vi "Byte177_188 (SubVI).vi"(2 "Channel Number":dbl, 3 "Input String":string) -> (0 "Output Lockout Status":bool, 1 "Output over current alert Ch I2T Levels":T1)   [LabVIEW 2024]
panel:
  in  "Channel Number 2":dbl
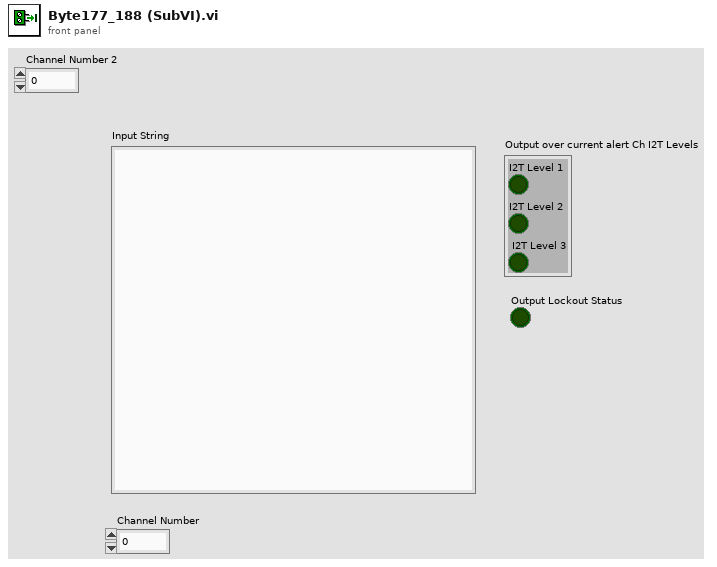
[diagram p1: front panel]
types:
  T1 = cluster{"I2T Level 1":bool, "I2T Level 2":bool, " I2T Level 3":bool}
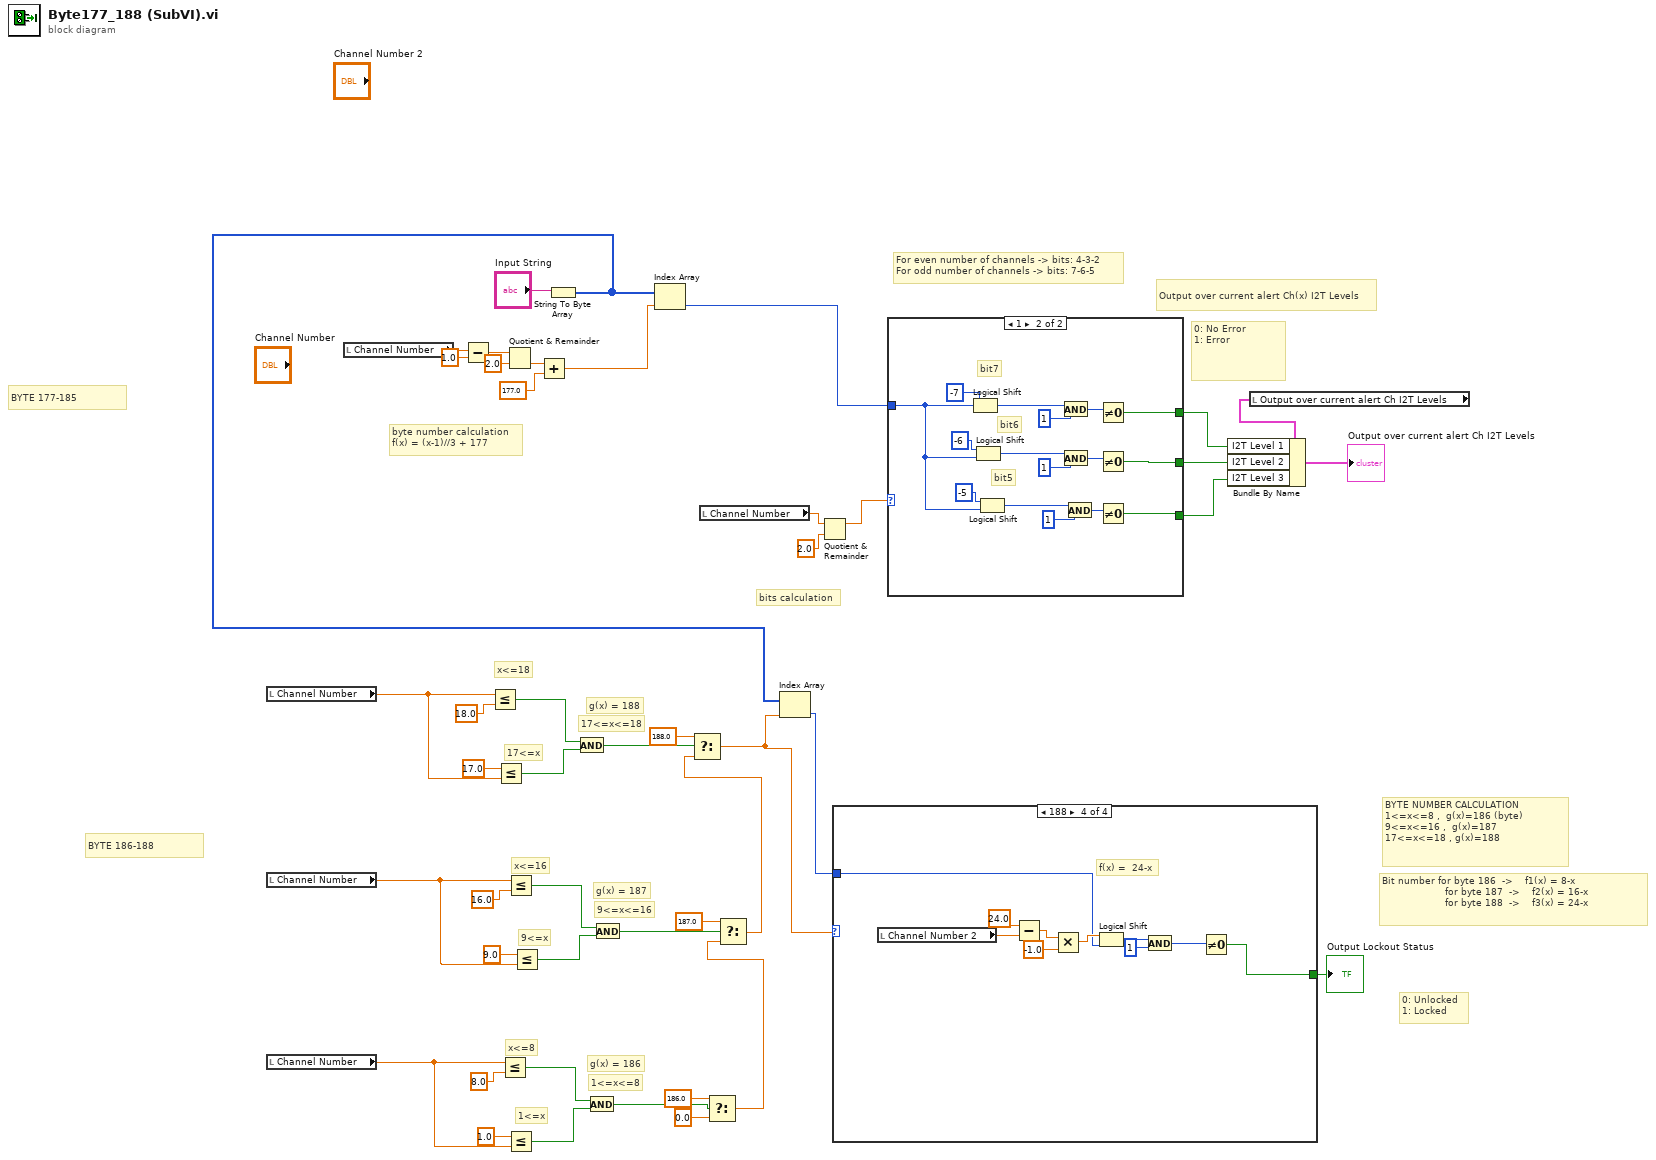
[diagram p0: block diagram]
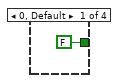
[diagram p2: hidden frame]
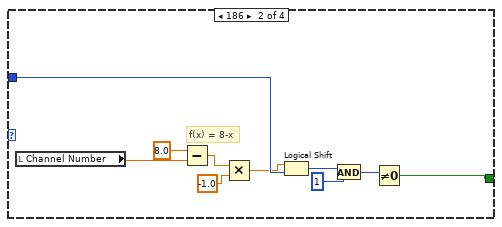
[diagram p3: hidden frame]
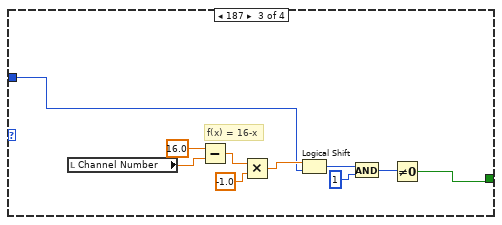
[diagram p4: hidden frame]
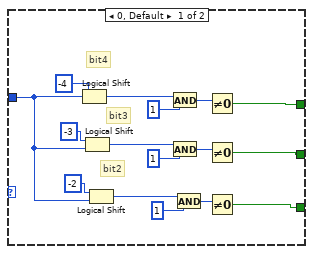
[diagram p5: hidden frame]
diagram:
  # "0: Unlocked\n1: Locked"
  # "BYTE 177-185"
  # "BYTE 186-188"
  # "Bit number for byte 186  ->    f1(x) = 8-x\n                     for byte 187  ->    f2(x) = 16-x\n                     for byte 188  ->    f3(x) = 24-x"
  # "BYTE NUMBER CALCULATION\n1<=x<=8 ,  g(x)=186 (byte)\n9<=x<=16 ,  g(x)=187\n17<=x<=18 , g(x)=188"
  # "g(x) = 186"
  # "1<=x<=8"
  # "1<=x"
  # "x<=8"
  # "g(x) = 187"
  # "g(x) = 188"
  # "9<=x<=16"
  # "9<=x"
  # "x<=16"
  # "17<=x<=18"
  # "17<=x"
  # "x<=18"
  # "byte number calculation\nf(x) = (x-1)//3 + 177"
  # "For even number of channels -> bits: 4-3-2\nFor odd number of channels -> bits: 7-6-5"
  # "0: No Error\n1: Error"
  # "Output over current alert Ch(x) I2T Levels"
  # "bits calculation"
  n1 = local read "Channel Number"() -> (w8:dbl)
  n2 = local read "Channel Number"() -> (w7:dbl)
  n3 = local read "Channel Number"() -> (w6:dbl)
  n4 = local read "Channel Number"() -> (w35:dbl)
  n5 = Subtract(x=w35, y=1.0) -> (x-y=w33:dbl)
  n6 = Less Or Equal?(x=w8, y=18.0) -> (x <= y?=w26:bool)
  n7 = Less Or Equal?(x=17.0, y=w8) -> (x <= y?=w25:bool)
  n8 = Less Or Equal?(x=w6, y=8.0) -> (x <= y?=w18:bool)
  n9 = Quotient & Remainder(x=w33, y=2.0) -> (floor(x/y)=w31:dbl)  [unwired: 1 out]
  n10 = Less Or Equal?(x=w7, y=16.0) -> (x <= y?=w22:bool)
  n11 = Less Or Equal?(x=1.0, y=w6) -> (x <= y?=w17:bool)
  n12 = Less Or Equal?(x=9.0, y=w7) -> (x <= y?=w21:bool)
  n13 = Add(x=w31, y=177.0) -> (x+y=w29:dbl)
  n14 = String To Byte Array(string="Input String") -> (unsigned byte array=w4:u8[])
  n15 = And(x=w26, y=w25) -> (x .and. y?=w16:bool)
  n16 = And(x=w18, y=w17) -> (x .and. y?=w14:bool)
  n17 = And(x=w22, y=w21) -> (x .and. y?=w15:bool)
  n18 = Index Array "Index Array"(array=w4, index=w29) -> (element=w41:u8)
  n19 = local read "Channel Number"() -> (w44:dbl)
  n20 = Select(t=186.0, s=w14, f=0.0) -> (s? t:f=w9:dbl)
  n21 = Select(t=187.0, s=w15, f=w9) -> (s? t:f=w5:dbl)
  n22 = Select(t=188.0, s=w16, f=w5) -> (s? t:f=w1:dbl)
  n23 = Index Array "Index Array"(array=w4, index=w1) -> (element=w2:u8)
  n24 = Quotient & Remainder(x=w44, y=2.0) -> (x-y*floor(x/y)=w42:dbl)  [unwired: 1 out]
  n25 = case shown="188" w1 {
    tunnel: w2 -> [_ w49 w57 w71]
    tunnel: [FALSE w50 w60 w67] -> w3
    frame 0, Default {
    }
    frame 186 {
      # "f(x) = 8-x"
      n26 = local read "Channel Number"() -> (w47:dbl)
      n27 = Subtract(x=8.0, y=w47) -> (x-y=w55:dbl)
      n28 = Multiply(x=w55, y=-1.0) -> (x*y=w48:dbl)
      n29 = Logical Shift(y=w48, x=w49) -> (x << y=w52:u8)
      n30 = And(x=w52, y=u8 1) -> (x .and. y?=w51:u8)
      n31 = Not Equal To 0?(x=w51) -> (x != 0?=w50:bool)
    }
    frame 187 {
      # "f(x) = 16-x"
      n32 = local read "Channel Number"() -> (w58:dbl)
      n33 = Subtract(x=16.0, y=w58) -> (x-y=w64:dbl)
      n34 = Multiply(x=w64, y=-1.0) -> (x*y=w59:dbl)
      n35 = Logical Shift(y=w59, x=w57) -> (x << y=w65:u8)
      n36 = And(x=w65, y=u8 1) -> (x .and. y?=w66:u8)
      n37 = Not Equal To 0?(x=w66) -> (x != 0?=w60:bool)
    }
    frame 188 {
      # "f(x) =  24-x"
      n38 = local read "Channel Number 2"() -> (w76:dbl)
      n39 = Subtract(x=24.0, y=w76) -> (x-y=w74:dbl)
      n40 = Multiply(x=w74, y=-1.0) -> (x*y=w72:dbl)
      n41 = Logical Shift(y=w72, x=w71) -> (x << y=w70:u8)
      n42 = And(x=w70, y=u8 1) -> (x .and. y?=w68:u8)
      n43 = Not Equal To 0?(x=w68) -> (x != 0?=w67:bool)
    }
  }
  "Output Lockout Status" <- w3
  n44 = case shown="1" w42 {
    tunnel: w41 -> [w80 w96]
    tunnel: [w79 w95] -> w39
    tunnel: [w78 w94] -> w40
    tunnel: [w77 w93] -> w38
    frame 0, Default {
      # "bit2"
      # "bit3"
      # "bit4"
      n45 = Logical Shift(y=i16 -4, x=w80) -> (x << y=w89:u8)
      n46 = Logical Shift(y=i16 -3, x=w80) -> (x << y=w85:u8)
      n47 = Logical Shift(y=i16 -2, x=w80) -> (x << y=w84:u8)
      n48 = And(x=w89, y=u8 1) -> (x .and. y?=w91:u8)
      n49 = And(x=w85, y=u8 1) -> (x .and. y?=w86:u8)
      n50 = And(x=w84, y=u8 1) -> (x .and. y?=w83:u8)
      n51 = Not Equal To 0?(x=w91) -> (x != 0?=w79:bool)
      n52 = Not Equal To 0?(x=w86) -> (x != 0?=w78:bool)
      n53 = Not Equal To 0?(x=w83) -> (x != 0?=w77:bool)
    }
    frame 1 {
      # "bit5"
      # "bit6"
      # "bit7"
      n54 = Logical Shift(y=i16 -7, x=w96) -> (x << y=w105:u8)
      n55 = Logical Shift(y=i16 -6, x=w96) -> (x << y=w101:u8)
      n56 = Logical Shift(y=i16 -5, x=w96) -> (x << y=w100:u8)
      n57 = And(x=w105, y=u8 1) -> (x .and. y?=w107:u8)
      n58 = And(x=w101, y=u8 1) -> (x .and. y?=w102:u8)
      n59 = And(x=w100, y=u8 1) -> (x .and. y?=w99:u8)
      n60 = Not Equal To 0?(x=w107) -> (x != 0?=w95:bool)
      n61 = Not Equal To 0?(x=w102) -> (x != 0?=w94:bool)
      n62 = Not Equal To 0?(x=w99) -> (x != 0?=w93:bool)
    }
  }
  n63 = local read "Output over current alert Ch I2T Levels"() -> (w37:T1)
  n64 = Bundle By Name(cluster=w37, "I2T Level 1"=w39, "I2T Level 2"=w40, "I2T Level 3"=w38) -> (→"Output over current alert Ch I2T Levels":T1)
